vi "Recieve Lockin Data.vi"(8 "error in (no error)":errorcluster, 11 "RP Lockin in":refnum<class "RP Transceiver.lvclass">) -> (0 "error out":errorcluster, 1 "Volatge out":cdb[](array[numeric]), 2 "Frequency out":dbl[](array[numeric]), 3 "RP Lockin out":refnum<class "RP Transceiver.lvclass">)   [LabVIEW 2015, in "RP Transceiver.lvclass"]
uses:
  RP Transceiver.lvclass
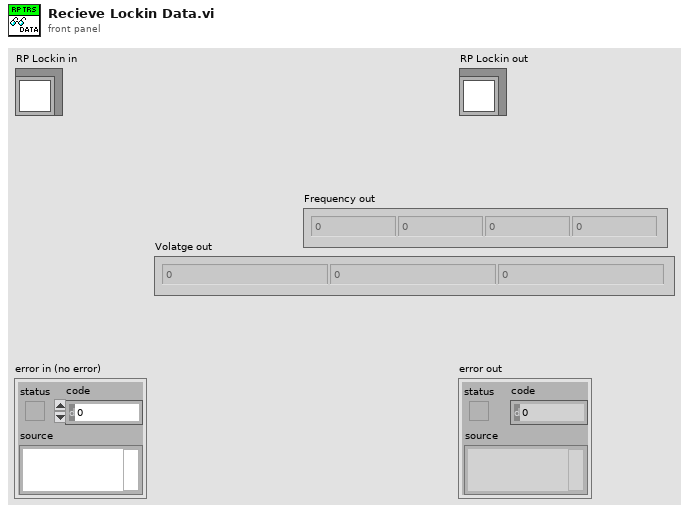
[diagram p1: front panel]
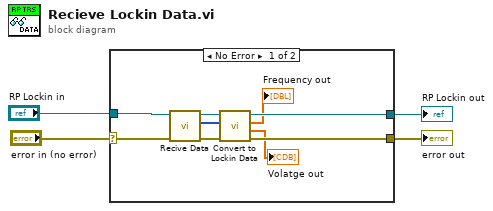
[diagram p0: block diagram]
diagram:
  n1 = case shown="No Error" "error in (no error)" {
    selector: "error in (no error)" -> [w13 w15]
    tunnel: [w10 w15] -> w3
    tunnel: [w11 w14] -> w1
    tunnel: "RP Lockin in" -> [w12 w14]
    frame No Error {
      n2 = call-dynamic "Recive Data.vi"("error in (no error)"=w13, "RP Transceiver in"=w12) -> ("error out"=w9:errorcluster, "Data out"=w8:i32[], "RP Transceiver out"=w5:refnum<class "RP Transceiver.lvclass">)  [unwired: 7 in]
      n3 = call-dynamic "Convert to Lockin Data.vi"("error in (no error)"=w9, "Raw data"=w8, "RP Lockin in"=w5) -> ("error out"=w10:errorcluster, "Volatge out"=→"Volatge out":cdb[], "Frequency out"=→"Frequency out":dbl[], "RP Lockin out"=w11:refnum<class "RP Transceiver.lvclass">)  [unwired: 5 in]
    }
    frame Error {
    }
  }
  "error out" <- w3
  "RP Lockin out" <- w1
